vi "subVi_Dialog_Double_Click.vi"() -> ()   [LabVIEW 2020]
doc: "This VI shows dialog window, which you can close by clicking the button \"OK, got it!\""
panel:
  in  "OK Button":bool
  # "Double click!"
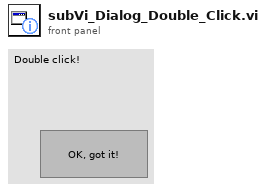
[diagram p1: front panel]
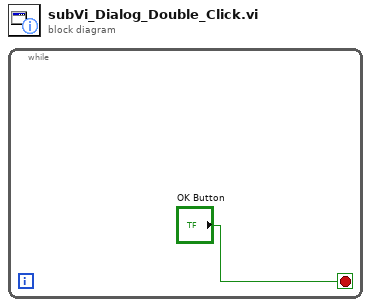
[diagram p0: block diagram]
diagram:
  n1 = while {
    stop <- "OK Button" stop-if-true
  }
